vi "range.vi"(9 "end":i32=10, 10 "step":i32=1, 11 "start":i32) -> (2 "range":i32[](array[numeric]))   [LabVIEW 2021]
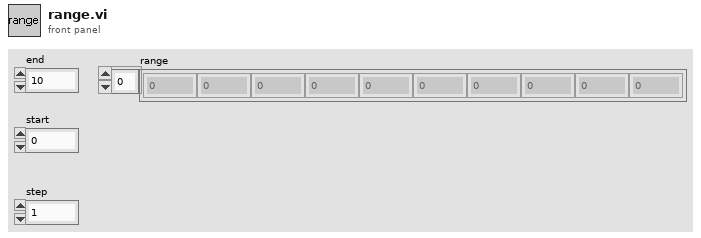
[diagram p1: front panel]
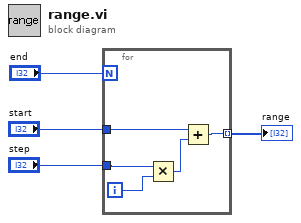
[diagram p0: block diagram]
diagram:
  n1 = for {
    N: "end" -> [_]
    tunnel: "start" -> [w9]
    tunnel: [w8] -> w1 mode=indexing
    tunnel: "step" -> [w5]
    i -> [w7]
    n2 = Multiply(x=w5, y=w7) -> (x*y=w6:i32)
    n3 = Add(x=w9, y=w6) -> (x+y=w8:i32)
  }
  "range" <- w1
